vi "Read Voltage Sweep.vi"(0 "VISA resource name":refnum<visa-resource-name>, 11 "error in (no error)":errorcluster) -> (4 "VISA resource name out":refnum<visa-resource-name>, 6 "Voltage Sweep Results":cluster{dbl[], dbl[]}(graph), 15 "error out":errorcluster)   [LabVIEW 2021, in "Keithley 648X Series.lvlib"]
doc: "Initiates the instrument, turns off zero check, and reads the fresh voltage sweep readings.\n\n<b>Note:</b>\nModel 6487 only"
uses:
  <instrlib>/Keithley 648X Series/Keithley 648X Series.lvlib
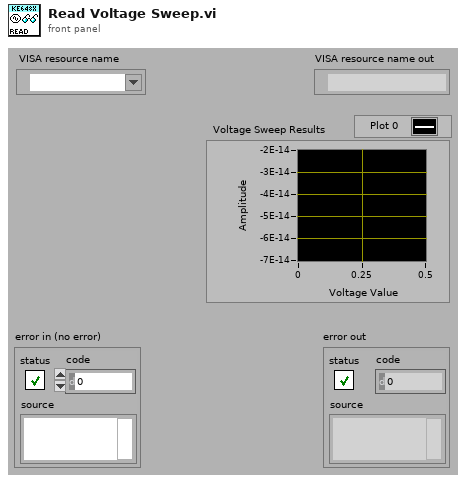
[diagram p1: front panel]
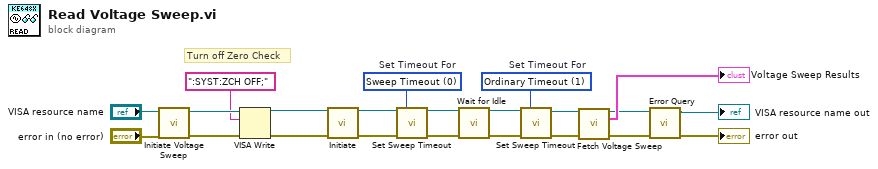
[diagram p0: block diagram]
diagram:
  w8 = u16 0 items=["Sweep Timeout", "Ordinary Timeout"]  # Set Timeout For
  w9 = u16 1 items=["Sweep Timeout", "Ordinary Timeout"]  # Set Timeout For
  # "Turn off Zero Check"
  n1 = call <instrlib>:"Initiate Voltage Sweep.vi"("error in (no error)"="error in (no error)", "VISA resource name"="VISA resource name") -> ("error out"=w4:errorcluster, "VISA resource name out"=w5:refnum<visa-resource-name>)  [unwired: 8 in]
  n2 = VISA Write(VISA resource name=w5, write buffer=":SYST:ZCH OFF;" ("format string"), error in (no error)=w4) -> (VISA resource name out=w2:refnum<visa-resource-name>, error out=w3:errorcluster)  [unwired: 1 out]
  n3 = call <instrlib>:"Initiate.vi"("VISA resource name"=w2, "error in (no error)"=w3) -> ("VISA resource name out"=w7:refnum<visa-resource-name>, "error out"=w6:errorcluster)  [unwired: 12 in]
  n4 = call <instrlib>:"Set Sweep Timeout.vi"("VISA resource name"=w7, "Set Timeout For (0: Sweep Timeout)"=w8, "error in (no error)"=w6) -> ("VISA resource name out"=w10:refnum<visa-resource-name>, "error out"=w11:errorcluster)  [unwired: 11 in]
  n5 = call <instrlib>:"Wait for Idle.vi"("VISA resource name"=w10, "error in (no error)"=w11) -> ("VISA resource name out"=w13:refnum<visa-resource-name>, "error out"=w12:errorcluster)  [unwired: 12 in]
  n6 = call <instrlib>:"Set Sweep Timeout.vi"("VISA resource name"=w13, "Set Timeout For (0: Sweep Timeout)"=w9, "error in (no error)"=w12) -> ("VISA resource name out"=w14:refnum<visa-resource-name>, "error out"=w15:errorcluster)  [unwired: 11 in]
  n7 = call <instrlib>:"Fetch Voltage Sweep.vi"("VISA resource name"=w14, "error in (no error)"=w15) -> ("VISA resource name out"=w17:refnum<visa-resource-name>, "Sweep Results"=→"Voltage Sweep Results":cluster{dbl[], dbl[]}, "error out"=w16:errorcluster)  [unwired: 11 in]
  n8 = call <instrlib>:"Error Query.vi"("error in (no error)"=w16, "VISA resource name"=w17) -> ("error out"=→"error out":errorcluster, "VISA resource name out"=→"VISA resource name out":refnum<visa-resource-name>)  [unwired: 6 in, 2 out]
